vi "onStart.vi"(8 "error in (no error)":errorcluster, 11 "MAUI":refnum<class "MAUI.lvclass">) -> (0 "error out":errorcluster, 3 "MAUI out":refnum<class "MAUI.lvclass">)   [LabVIEW 2016, in "MAUI.lvclass"]
doc: "JKI State Machine Objects (SMO) 1.3.0.56\nJKI - JKI\nCopyright (c) 2017, JKI"
uses:
  MAUI.lvclass
  <vilib>/Levylab/Embedded SMO UI/EmbeddedSMO.lvclass
  C:/Program Files (x86)/National Instruments/LabVIEW 2016/vi.lib/JKI/JKI SMO/SMO/SMO.lvclass
  MAUI.lvclass/MAUI.ctl
  <vilib>/JKI/JKI SMO/SMO.UI/SMO.UI.lvclass
  <vilib>/JKI/JKI SMO/SMO/SMO.lvclass
panel:
  # "For instructions on how to use the JKI State Machine Objects, examples and video tutorials, visit:\nhttp://jki.net/state-machine-objects/\n\nJKI State Machine Objects™\nhttp://jki.net/state-machine-objects/\nCopyright (C) 2005-2015, JKI <info@jki.net>\nALL RIGHTS RESERVED"
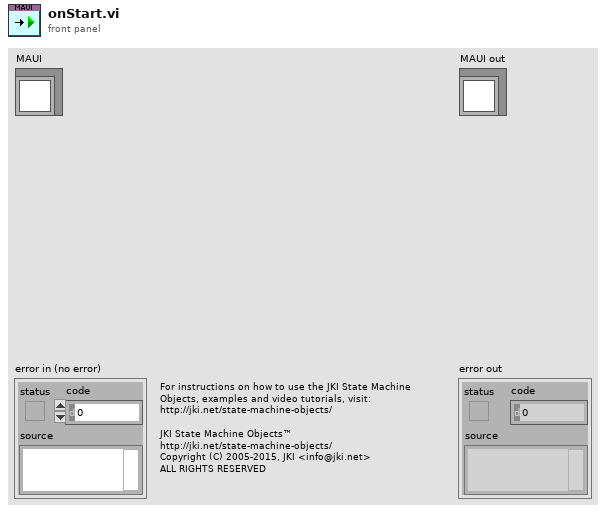
[diagram p1: front panel]
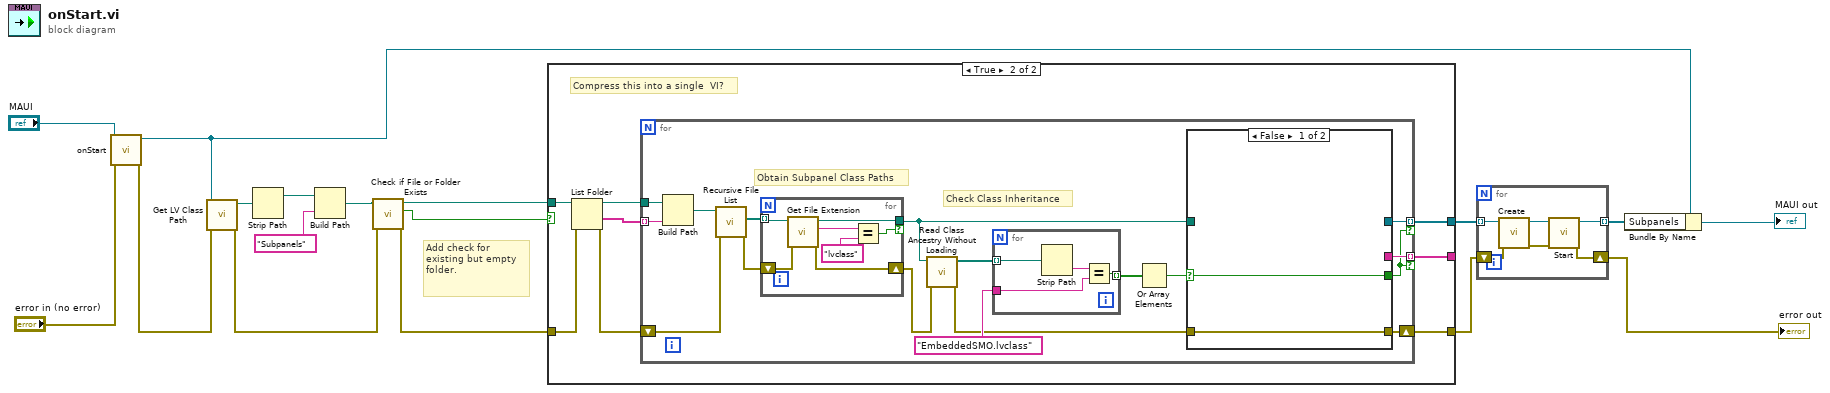
[diagram p0: block diagram]
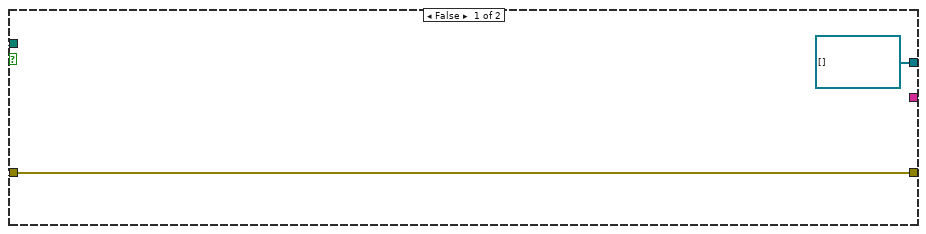
[diagram p2: hidden frame]
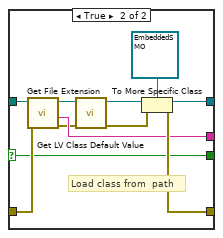
[diagram p3: hidden frame]
diagram:
  # "Add check for existing but empty folder."
  n1 = call-parent "onStart.vi"("error in (no error)"="error in (no error)", "SMO"="MAUI") -> ("error out"=w9:errorcluster, "SMO out"=w2:refnum<class "MAUI.lvclass">)  [unwired: 8 in]
  n2 = call <vilib>:"Get LV Class Path.vi"("error in (no error)"=w9, "object"=w2) -> ("error out"=w10:errorcluster, "class path"=w17:path)  [unwired: 8 in]
  n3 = Strip Path(path=w17) -> (stripped path=w16:path)  [unwired: 1 out]
  n4 = Build Path(base path=w16, name or relative path="Subpanels") -> (appended path=w14:path)
  n5 = call <vilib>:"Check if File or Folder Exists.vi"("error in (no error)"=w10, "path"=w14) -> ("error out"=w12:errorcluster, "file or folder exists?"=w11:bool, "dup path"=w13:path)  [unwired: 7 in]
  n6 = case shown="True" w11 {
    tunnel: w13 -> [w20 w28]
    tunnel: w12 -> [w19 w23]
    tunnel: [w19 w22] -> w7
    tunnel: [refnum<class "EmbeddedSMO.lvclass">[] [] w24] -> w8
    tunnel: [_ w21] -> _
    frame False {
      n7 = Create Folder(path (use dialog)=w20, error in=w19) -> ()  [unwired: 1 in, 3 out]
    }
    frame True {
      # "Compress this into a single  VI?"
      n8 = List Folder(path=w28, error in=w23) -> (path out=w27:path, folder names=w26:string[], error out=w25:errorcluster)  [unwired: 2 in, 1 out]
      n9 = for {
        tunnel: w27 -> [w45]
        tunnel: w26 -> [w44] mode=indexing
        tunnel: [w40] -> w24 mode=indexing if=w29
        shift-right: [w32] -> w22
        shift-left: w25 -> [w36]
        tunnel: [w30] -> w21 mode=indexing if=w29
        # "Check Class Inheritance"
        # "Obtain Subpanel Class Paths"
        n10 = Build Path(base path=w45, name or relative path=w44) -> (appended path=w43:path)
        n11 = call <vilib>:"Recursive File List.vi"("error in (no error)"=w36, "Folder Path"=w43) -> ("error out"=w35:errorcluster, "All Files in Dir"=w42:path[])  [unwired: 5 in, 3 out]
        n12 = for {
          tunnel: w42 -> [w67] mode=indexing
          tunnel: [w66] -> w41 if=w65
          shift-right: [w63] -> w34
          shift-left: w35 -> [w64]
          n13 = call <vilib>:"Get File Extension.vi"("error in (no error)"=w64, "file"=w67) -> ("error out"=w63:errorcluster, "lowercase file extension"=w69:string, "dup file"=w66:path)  [unwired: 5 in, 2 out]
          n14 = Equal?(x=w69, y="lvclass") -> (x = y?=w65:bool)
        }
        n15 = call <vilib>:"Read Class Ancestry Without Loading.vi"("error in (no error)"=w34, "LabVIEW Class Path"=w41) -> ("error out"=w33:errorcluster, "Class Ancestry"=w39:path[])  [unwired: 8 in]
        n16 = for {
          tunnel: w39 -> [w62] mode=indexing
          tunnel: [w60] -> w38 mode=indexing
          tunnel: "EmbeddedSMO.lvclass" -> [w59]
          n17 = Strip Path(path=w62) -> (name=w61:string)  [unwired: 1 out]
          n18 = Equal?(x=w61, y=w59) -> (x = y?=w60:bool)
        }
        n19 = Or Array Elements(Boolean array=w38) -> (logical OR=w31:bool)
        n20 = case shown="False" w31 {
          selector: w31 -> [w46 w48]
          tunnel: w41 -> [_ w53]
          tunnel: [_ w58] -> w40
          tunnel: w33 -> [w47 w50]
          tunnel: [w47 w54] -> w32
          tunnel: [_ w51] -> w30
          tunnel: [w46 w48] -> w29
          frame False {
          }
          frame True {
            # "Load class from  path"
            n21 = call <vilib>:"Get File Extension.vi"("error in (no error)"=w50, "file"=w53) -> ("error out"=w49:errorcluster, "filename without extension"=w51:string, "dup file"=w52:path)  [unwired: 5 in, 2 out]
            n22 = call <vilib>:"Get LV Class Default Value.vi"("error in (no error)"=w49, "class path"=w52) -> ("error out"=w55:errorcluster, "object"=w57:refnum<class>)  [unwired: 8 in]
            n23 = To More Specific Class(target class=refnum<class "EmbeddedSMO.lvclass"> refnum ("EmbeddedSMO"), reference=w57, error in=w55) -> (specific class reference=w58:refnum<class "EmbeddedSMO.lvclass">, error out=w54:errorcluster)
          }
        }
      }
    }
  }
  n24 = for {
    tunnel: w8 -> [w75] mode=indexing
    tunnel: [w74] -> w3 mode=indexing
    shift-right: [w70] -> w4
    shift-left: w7 -> [w71]
    n25 = call <vilib>:"Create.vi"("error in (no error)"=w71, "SMO"=w75) -> ("error out"=w72:errorcluster, "SMO out"=w73:refnum<class "EmbeddedSMO.lvclass">)  [unwired: 7 in, 1 out]
    n26 = call <vilib>:"Start.vi"("error in (no error)"=w72, "SMO"=w73) -> ("error out"=w70:errorcluster, "SMO out"=w74:refnum<class "EmbeddedSMO.lvclass">)  [unwired: 8 in]
  }
  "error out" <- w4
  n27 = Bundle By Name(cluster=w2, "Subpanels"=w3) -> (→"MAUI out":refnum<class "MAUI.lvclass">)
